vi "disable deco strings.vi"(8 "error in (no error)":errorcluster) -> (0 "error out":errorcluster)   [LabVIEW 2012]
uses:
  <vilib>/regexp/Match Regular Expression.xnode
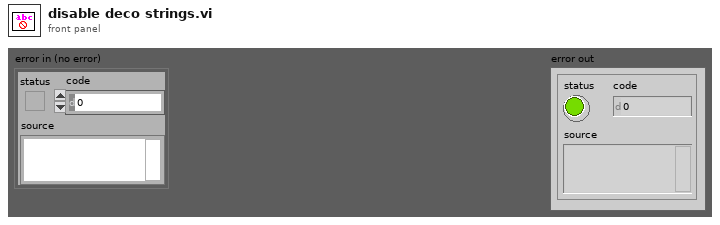
[diagram p1: front panel]
types:
  T1 = enum8{"Enabled", "Disabled", "Disabled and Grayed Out"}
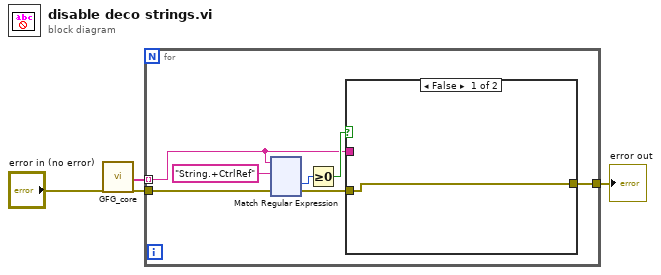
[diagram p0: block diagram]
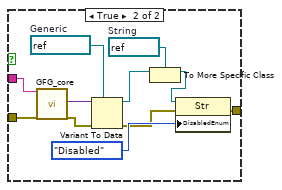
[diagram p2: hidden frame]
diagram:
  n1 = call "GFG_core.vi"("error in (no error)"="error in (no error)") -> ("All Variable Names Out"=w4:string[], "error out"=w3:errorcluster)  [unwired: 12 in, 5 out]
  n2 = for {
    tunnel: w4 -> [w8] mode=indexing
    tunnel: w3 -> [w7]
    tunnel: [w5] -> w1
    n3 = xnode "Match Regular Expression"("input string"=w8, "regular expression"="String.+CtrlRef", "error in"=w7) -> ("offset past match"=w9:i32, "error out"=w6:errorcluster)  [unwired: 3 in, 3 out]
    n4 = Greater Or Equal To 0?(x=w9) -> (x >= 0?=w10:bool)
    n5 = case shown="False" w10 {
      tunnel: w8 -> [_ w23]
      tunnel: w6 -> [w12 w20]
      tunnel: [w12 w13] -> w5
      frame False {
      }
      frame True {
        w19 = refnum<vi> refnum  # Generic
        w17 = refnum<vi> refnum  # String
        n6 = call "GFG_core.vi"("Variable Name in"=w23, "error in (no error)"=w20) -> ("Variant Out"=w22:variant, "error out"=w15:errorcluster)  [unwired: 11 in, 5 out]
        n7 = Variant To Data(error in=w15, type=w19, Variant=w22) -> (data=w18:refnum<vi>, error out=w14:errorcluster)
        n8 = To More Specific Class(target class=w17, reference=w18) -> (specific class reference=w16:refnum<vi>)  [unwired: 1 in, 1 out]
        n9 = property class="Str"(reference=w16, error in=w14, "DisabledEnum"=T1."Disabled" ("Disabled")) -> (error out=w13:errorcluster)  [unwired: 1 out]
      }
    }
  }
  "error out" <- w1
